vi "Main.vi"() -> ()   [LabVIEW 2013]
uses:
  <vilib>/Instr/_visa.llb/VISA Configure Serial Port (Instr).vi
panel:
  out "수신":string
  out "바이트":u32
  in  "VISA 리소스 이름":refnum<visa-resource-name>="COM3"
  out "동작 입력":string
  out "Motor Pos C":i32
  out "Motor Pos R":i32
  out "Motor Pos L":i32
  out "Motor Axis":string
  in  "Servo":bool
  out "Serial Error Out":errorcluster caption="시리얼 에러 출력"
  in  "Serial Error In":errorcluster caption="시리얼 에러 입력"
  in  "통신속도":u32(ring)=1 items=["4800", "9600", "19200", "38400", "57600", "115200"]
  out "C Motor Work":string
  out "R Motor Work":string
  out "L Motor Work":string
  in  "Encoder RESET":bool
  in  "FULL DOWN":bool
  in  "FULL UP":bool
  out "제어 상태":string="비상제어"
  in  "수동 모터 C":i32(slide)=127 scale=0.0..256.0
  in  "수동 모터 R":i32(slide)=127 scale=0.0..256.0
  in  "수동 모터 L":i32(slide)=127 scale=0.0..256.0
  in  "네트워크 선택":string(combo)="오프라인"
  in  "제어":string(combo)="비상제어"
  in  "정지 버튼":bool
  out "Game Pos C":i32=127
  out "Game Pos R":i32=127
  out "Game Axis":string
  out "Game Pos L":i32=127
  out "UDP Error Out":errorcluster caption="UDP 에러 출력"
  in  "UDP Error In":errorcluster caption="UDP 에러 입력"
  in  "IP":string="127.0.0.1"
  in  "PORT":u16=50
  out "네트워크 상태":string="OFFLINE"
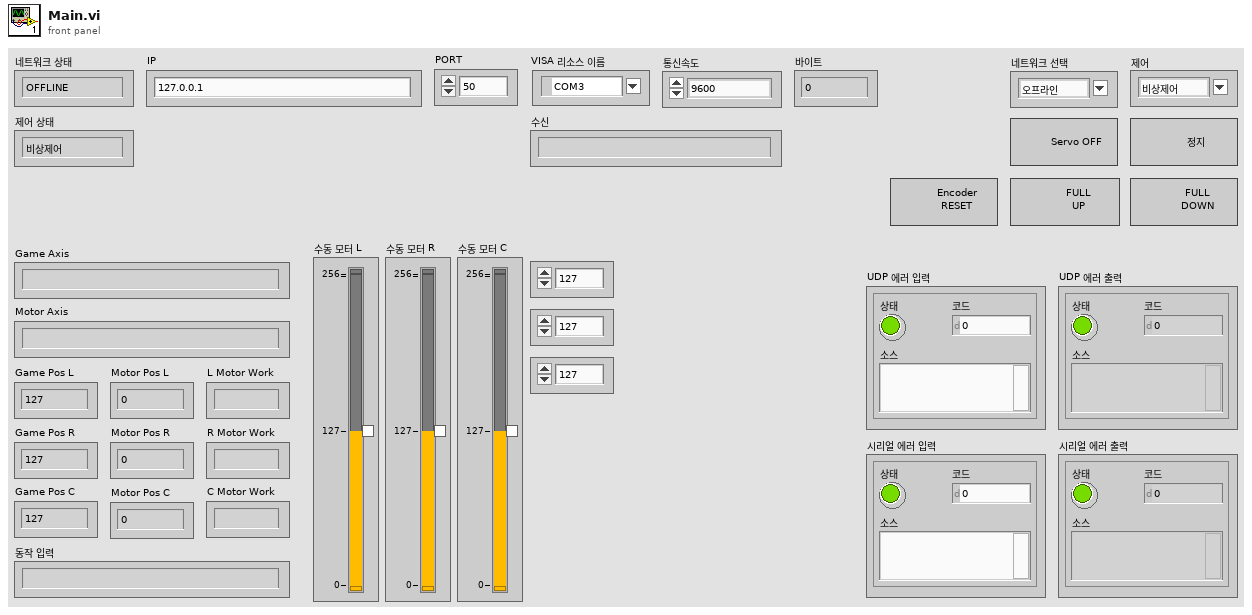
[diagram p1: front panel]
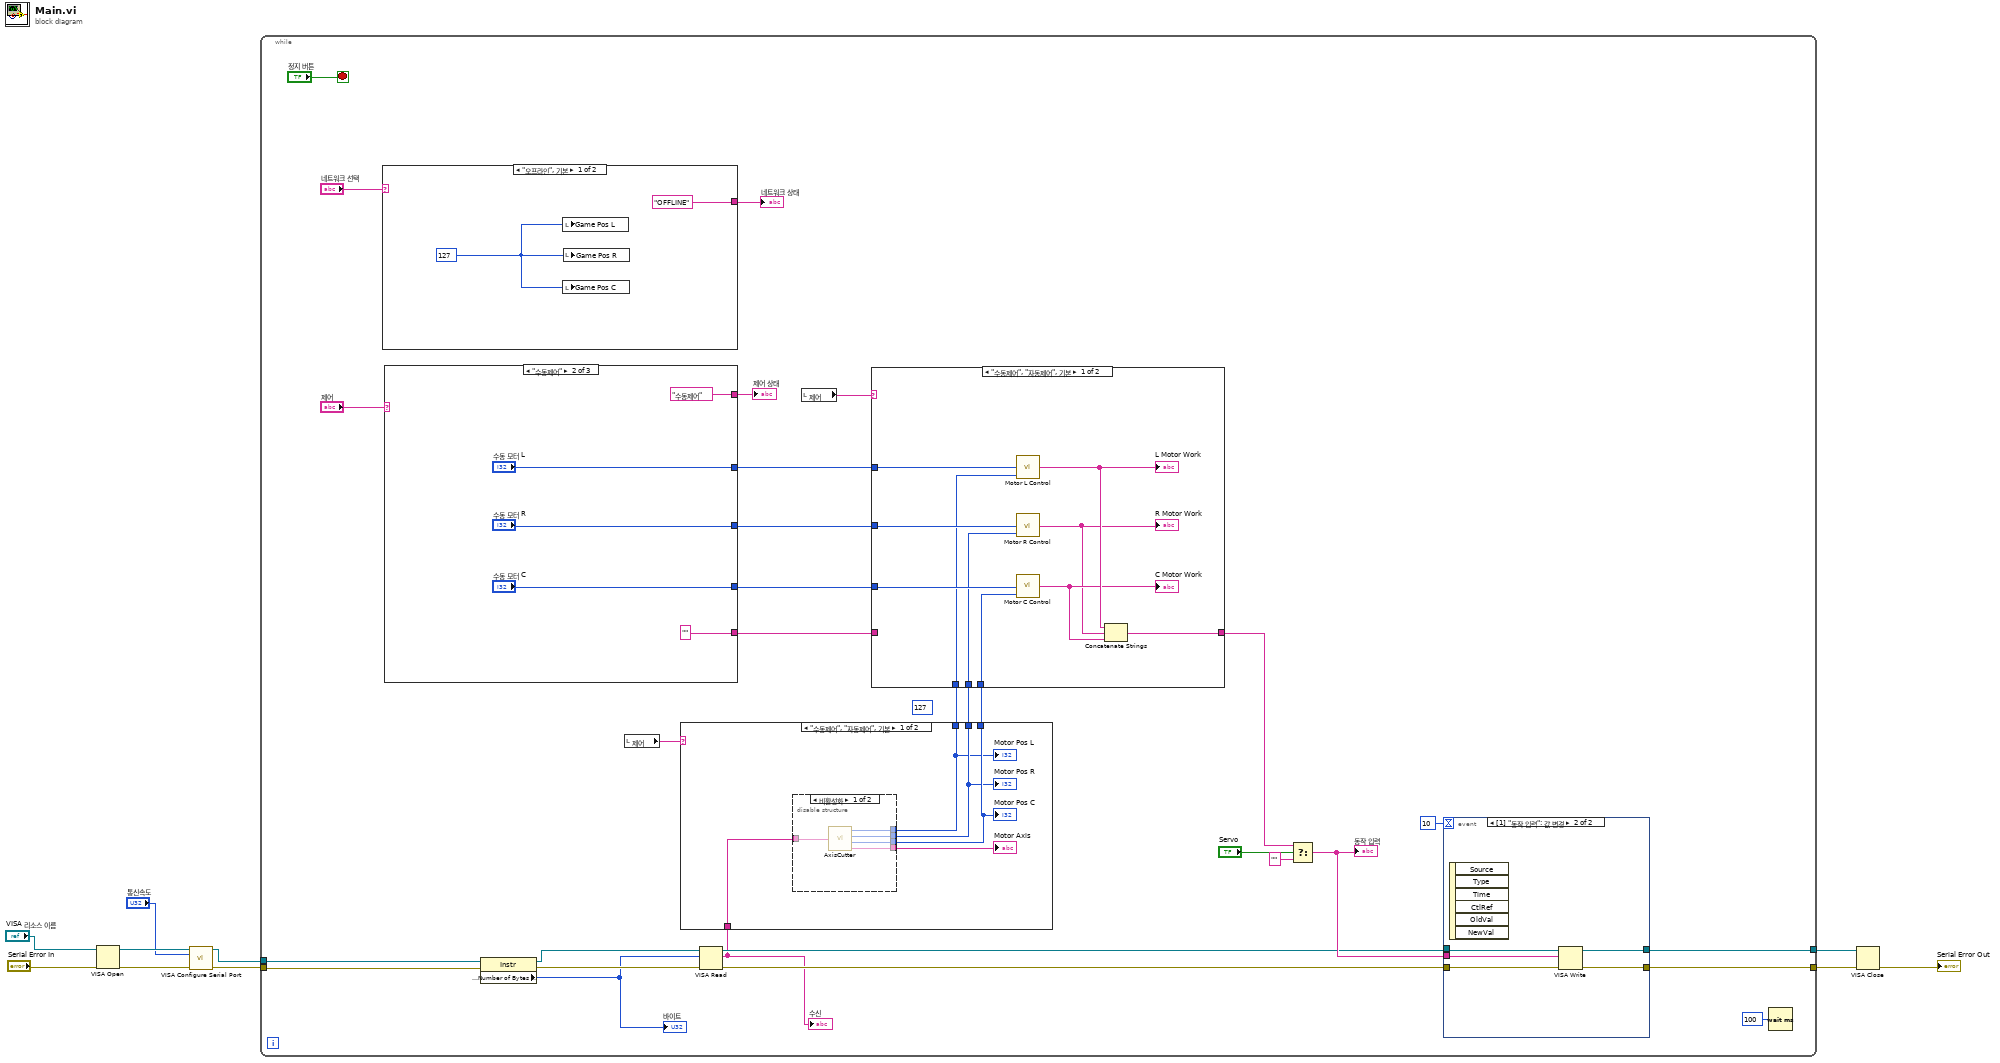
[diagram p0: block diagram]
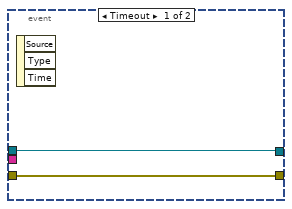
[diagram p2: hidden frame]
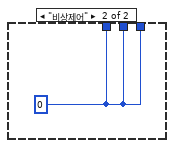
[diagram p4: hidden frame]
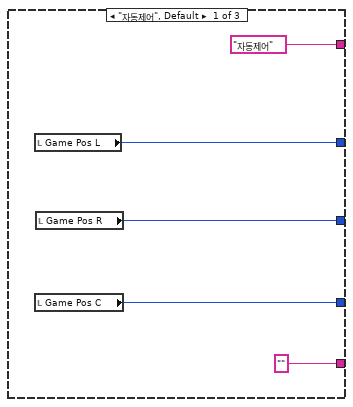
[diagram p6: hidden frame]
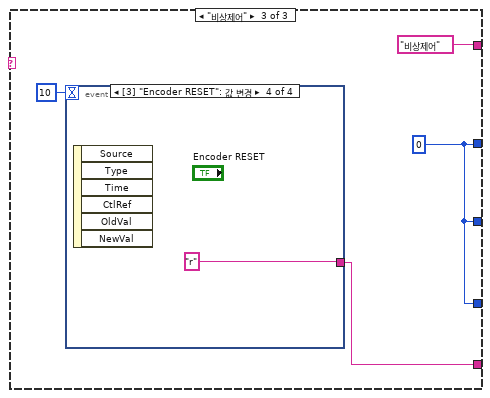
[diagram p7: hidden frame]
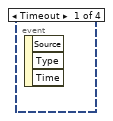
[diagram p8: hidden frame]
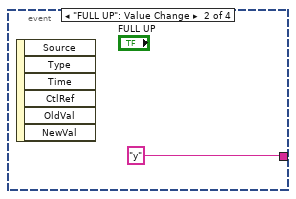
[diagram p9: hidden frame]
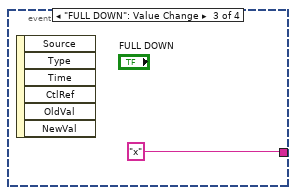
[diagram p10: hidden frame]
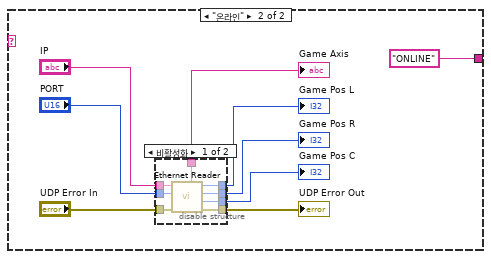
[diagram p11: hidden frame]
diagram:
  n1 = VISA Open(error in (no error)="Serial Error In", VISA resource name="VISA 리소스 이름") -> (VISA resource name=w4:refnum<visa-resource-name>, error out=w7:errorcluster)  [unwired: 3 in]
  n2 = call-poly "VISA Configure Serial Port"("VISA resource name"=w4, "baud rate (9600)"="통신속도", "error in (no error)"=w7) -> ("VISA resource name out"=w5:refnum<visa-resource-name>, "error out"=w6:errorcluster)  [unwired: 11 in]
  n3 = while {
    tunnel: [w21] -> w9
    tunnel: [w20] -> w8
    tunnel: w6 -> [w19]
    tunnel: w5 -> [w18]
    stop <- "정지 버튼" stop-if-true
    (unwired) 127
    n4 = case "케이스 구조" shown="\"오프라인\", 기본" "네트워크 선택" {
      tunnel: ["OFFLINE" "ONLINE"] -> w40
      frame "오프라인", Default {
        w87 = 127
        n5 = local write "Game Pos L"(w87) -> ()
        n6 = local write "Game Pos C"(w87) -> ()
        n7 = local write "Game Pos R"(w87) -> ()
      }
      frame "온라인" {
        n8 = disable-structure shown="비활성화" {
          disable-tunnel: "UDP Error In" -> [w105 _]
          disable-tunnel: [w104 _] -> w96
          disable-tunnel: "PORT" -> [w103 _]
          disable-tunnel: "IP" -> [w102 _]
          disable-tunnel: [w101 _] -> w93
          disable-tunnel: [w100 _] -> w92
          disable-tunnel: [w99 _] -> w91
          disable-tunnel: [w98 _] -> w90
          frame Disabled {
            n9 = call "Ethernet Reader.vi"("IP"=w102, "포트"=w103, "에러 입력(에러 없음)"=w105) -> ("Axis"=w101:string, "L"=w100:i32, "R"=w99:i32, "C"=w98:i32, "에러 출력"=w104:errorcluster)  [unwired: 2 in]
          }
          frame Enabled {
          }
        }
        "UDP Error Out" <- w96
        "Game Pos R" <- w91
        "Game Pos C" <- w90
        "Game Pos L" <- w92
        "Game Axis" <- w93
      }
    }
    "네트워크 상태" <- w40
    n10 = case shown="\"수동제어\"" "제어" {
      tunnel: [w74 "수동 모터 C" w83] -> w31
      tunnel: [w73 "수동 모터 R" w83] -> w32
      tunnel: [w72 "수동 모터 L" w83] -> w33
      tunnel: ["자동제어" "수동제어" "비상제어"] -> w36
      tunnel: ["" "" w80] -> w34
      frame "자동제어", Default {
        n11 = local read "Game Pos L"() -> (w72:i32)
        n12 = local read "Game Pos C"() -> (w74:i32)
        n13 = local read "Game Pos R"() -> (w73:i32)
      }
      frame "수동제어" {
      }
      frame "비상제어" {
        w83 = 0
        n14 = event shown="[3] \"Encoder RESET\": 값 변경" {
          selector: _ -> [_ _ _ _]
          dyn-events: _ -> [_ _ _ _]
          timeout: 10 -> [_ _ _ _]
          tunnel: [_ "y" "x" "r"] -> w80
          event Timeout {
            n15 = event-data() -> ()  [unwired: 1 in, 3 out]
          }
          event "FULL UP": Value Change {
            n16 = event-data() -> ()  [unwired: 1 in, 6 out]
          }
          event "FULL DOWN": Value Change {
            n17 = event-data() -> ()  [unwired: 1 in, 6 out]
          }
          event "Encoder RESET": Value Change {
            n18 = event-data() -> ()  [unwired: 1 in, 6 out]
          }
        }
      }
    }
    "제어 상태" <- w36
    n19 = property class="Instr"(reference=w18, error in=w19) -> (reference out=w15:refnum<visa-resource-name>, error out=w17:errorcluster, "Serial Settings:Number of Bytes at Serial Port"=w13:u32)
    "바이트" <- w13
    n20 = local read "제어"() -> (w30:string)
    n21 = VISA Read(VISA resource name=w15, byte count=w13, error in (no error)=w17) -> (VISA resource name out=w14:refnum<visa-resource-name>, read buffer=w12:string, error out=w16:errorcluster)  [unwired: 1 out]
    "수신" <- w12
    n22 = case shown="\"수동제어\", \"자동제어\", 기본" w30 {
      tunnel: [w49 w58] -> w24
      tunnel: [w50 w58] -> w23
      tunnel: [w51 w58] -> w22
      tunnel: w12 -> [w48 _]
      frame "수동제어", "자동제어", Default {
        n23 = disable-structure shown="비활성화" {
          disable-tunnel: w48 -> [w57 _]
          disable-tunnel: [w56 _] -> w52
          disable-tunnel: [w55 _] -> w51
          disable-tunnel: [w54 _] -> w50
          disable-tunnel: [w53 _] -> w49
          frame Disabled {
            n24 = call "AxisCutter.vi"("수신"=w57) -> ("L"=w53:i32, "R"=w54:i32, "C"=w55:i32, "Axis"=w56:string)
          }
          frame Enabled {
          }
        }
        "Motor Axis" <- w52
        "Motor Pos L" <- w49
        "Motor Pos R" <- w50
        "Motor Pos C" <- w51
      }
      frame "비상제어" {
        w58 = 0
      }
    }
    n25 = local read "제어"() -> (w35:string)
    n26 = case shown="\"수동제어\", \"자동제어\", 기본" w35 {
      tunnel: w34 -> [_ w69]
      tunnel: w33 -> [w67 _]
      tunnel: w32 -> [w65 _]
      tunnel: w31 -> [w66 _]
      tunnel: [w68 w69] -> w28
      tunnel: w24 -> [w64 _]
      tunnel: w23 -> [w63 _]
      tunnel: w22 -> [w62 _]
      frame "수동제어", "자동제어", Default {
        n27 = call "Motor L Control.vi"("Motor Axis Pos"=w64, "Game Axis Pos"=w67) -> ("Motor Move"=w61:string)  [unwired: 1 in]
        "L Motor Work" <- w61
        n28 = call "Motor R Control.vi"("Motor Axis Pos"=w63, "Game Axis Pos"=w65) -> ("Motor Move"=w59:string)  [unwired: 1 in]
        "R Motor Work" <- w59
        n29 = call "Motor C Control.vi"("Motor Axis Pos"=w62, "Game Axis Pos"=w66) -> ("Motor Move"=w60:string)  [unwired: 1 in]
        "C Motor Work" <- w60
        n30 = Concatenate Strings(w61, w59, w60) -> (w68:string)
      }
      frame "비상제어" {
      }
    }
    n31 = Select(t=w28, s="Servo", f="") -> (s? t:f=w25:string)
    "동작 입력" <- w25
    n32 = event shown="[1] \"동작 입력\": 값 변경" {
      selector: _ -> [_ _]
      dyn-events: _ -> [_ _]
      timeout: 10 -> [_ _]
      tunnel: [w42 w47] -> w20
      tunnel: [w41 w46] -> w21
      tunnel: w25 -> [_ w45]
      tunnel: w16 -> [w41 w44]
      tunnel: w14 -> [w42 w43]
      event Timeout {
        n33 = event-data() -> ()  [unwired: 1 in, 3 out]
      }
      event "동작 입력": Value Change {
        n34 = event-data() -> ()  [unwired: 1 in, 6 out]
        n35 = VISA Write(VISA resource name=w43, write buffer=w45, error in (no error)=w44) -> (VISA resource name out=w47:refnum<visa-resource-name>, error out=w46:errorcluster)  [unwired: 1 out]
      }
    }
    n36 = Wait (ms)(milliseconds to wait=u32 100 ("대기 시간(ms)")) -> ()  [unwired: 1 out]
  }
  n37 = VISA Close(VISA resource name=w8, error in (no error)=w9) -> (error out=→"Serial Error Out":errorcluster)
